vi "requestStatus.vi"(8 "error in (no error)":errorcluster, 11 "MonoCommunicator in":refnum<class "MonoCommunicator.lvclass">) -> (0 "error out":errorcluster, 3 "MonoCommunicator out":refnum<class "MonoCommunicator.lvclass">)   [LabVIEW 2016, in "MonoCommunicator.lvclass"]
uses:
  MonoCommunicator.lvclass
  MonoCommunicator.lvclass/MonoCommunicator.ctl
  MonoPubSubData/MonoPubSubData.lvclass/MonoPubSubData.ctl
  MonoPubSubData/MonoPubSubData.lvclass
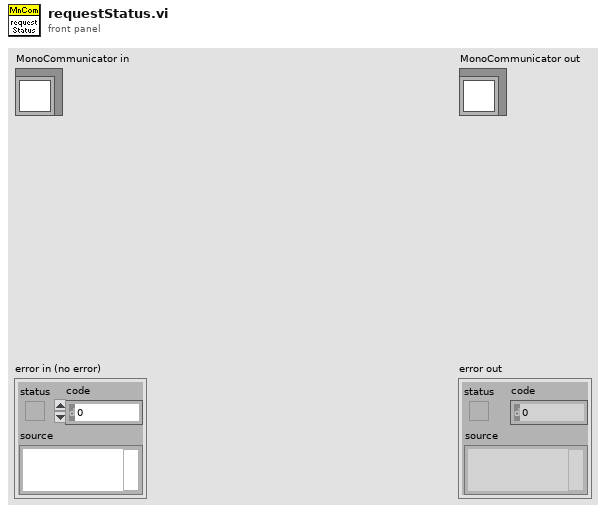
[diagram p1: front panel]
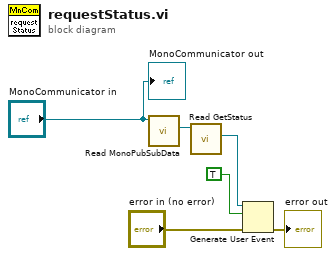
[diagram p0: block diagram]
diagram:
  n1 = call "Read MonoPubSubData.vi"("MonoCommunicator in"="MonoCommunicator in") -> ("MonoPubSubData.lvclass"=w1:refnum<class "MonoPubSubData.lvclass">)  [unwired: 8 in, 2 out]
  n2 = call "Read GetStatus.vi"("MonoPubSubData in"=w1) -> ("GetStatus"=w5:refnum<user-event>)  [unwired: 8 in, 2 out]
  n3 = Generate User Event(user event=w5, event data cluster=TRUE ("event data"), error in="error in (no error)") -> (error out=→"error out":errorcluster)  [unwired: 1 in, 1 out]
  "MonoCommunicator out" <- "MonoCommunicator in"
